vi "Module - Page Report.vi"(11 "Stop":bool) -> ()   [LabVIEW 2020]
uses:
  Control/State - eFGV.ctl
panel:
  in  "header name":T1={"Value 1"="", "Datetime"="Datetime", "Test Number"="Test Number", "Chart No"="Chart No", "Test Cycle"="Test Cycle", "Order Number"="Order Number", "Work Station"="Work Station", "Test Catergory"="Test Catergory", "Test Type"="Test Type", "Tested by"="Tested by", "Test Status"="Test Status", "Approved by TPI"="Approved by TPI"}
  in  "Table Report":T2(array[cluster])
  in  "Search 2":bool
  in  "Test Cycle":string(combo)
  in  "Test Type":string(combo)
  in  "Test Number":u16
  in  "Work Station":string(combo)
  in  "End Date":timestamp caption="To" format="%<%x %.3X>T"
  in  "Start Date":timestamp caption="Date" format="%<%x %.3X>T"
  in  "TPI Approval":bool
  in  "Overall Test Status":bool
  in  "Selection":string(combo)
  in  "Report Type":string(combo)
  # "REPORT"
  # "Approved Only"
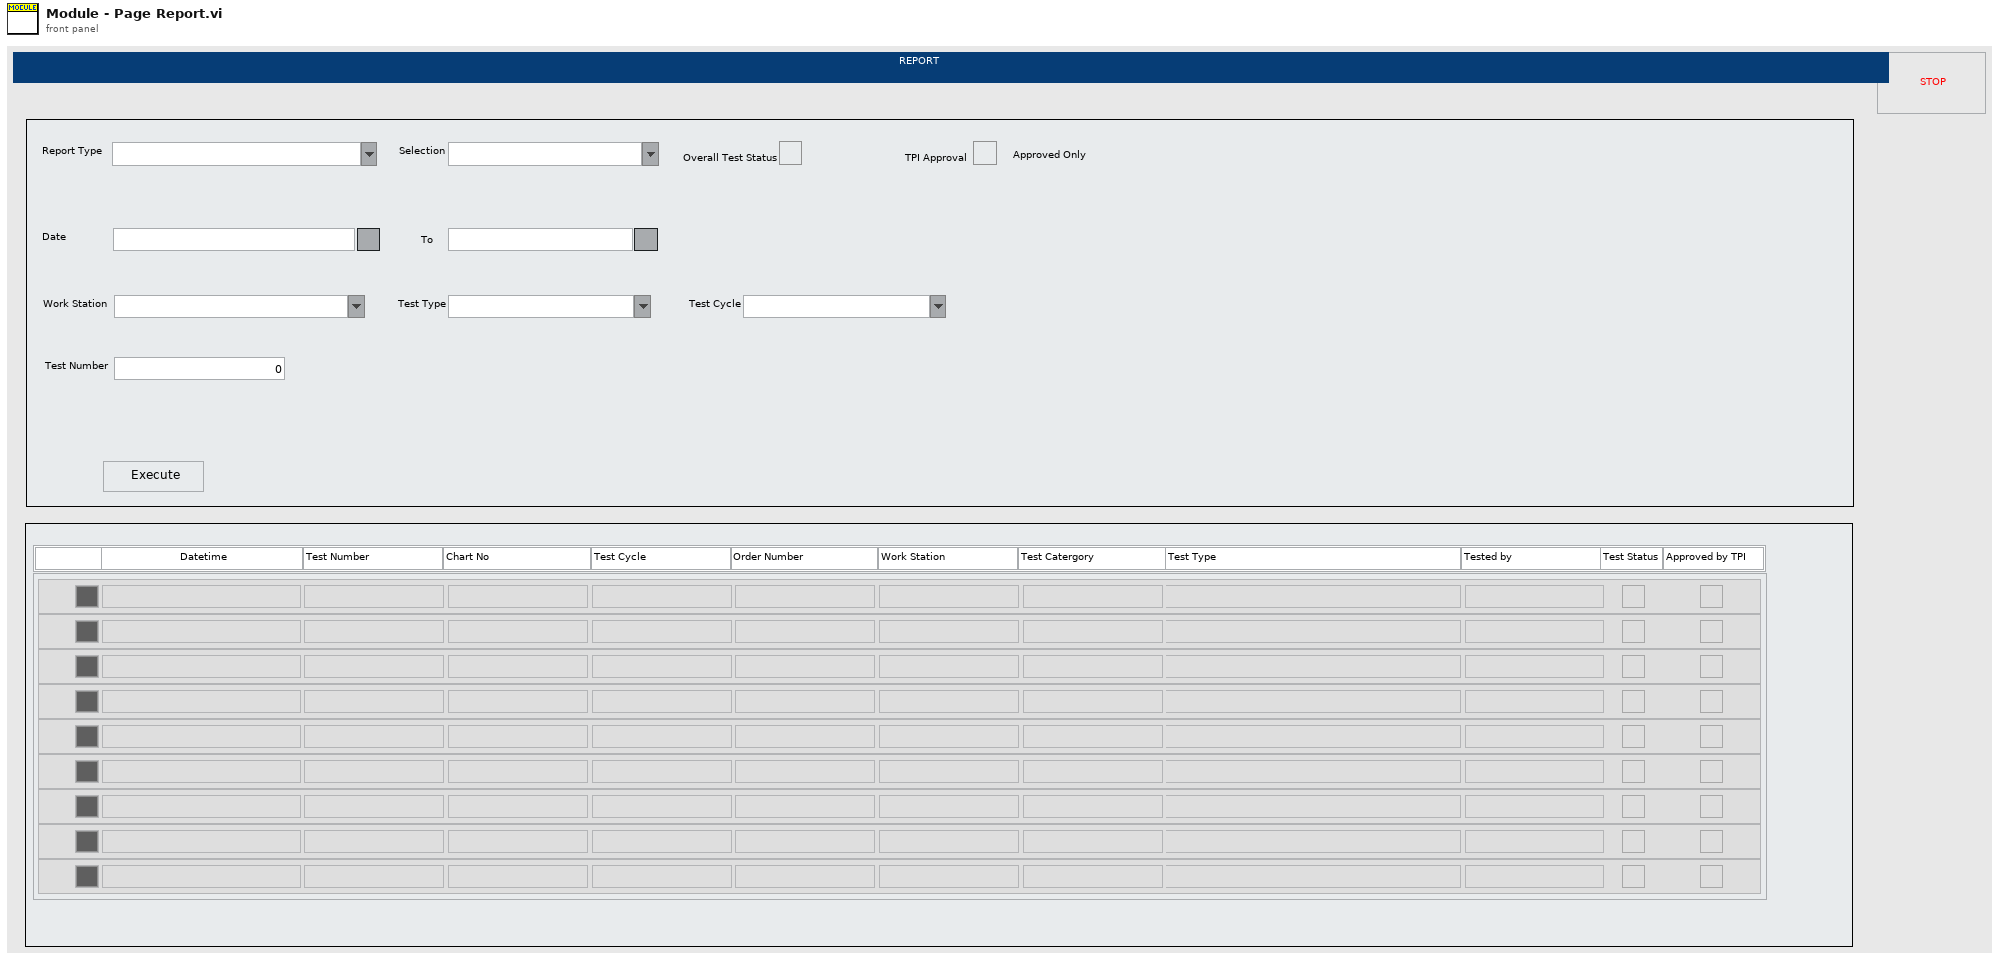
[diagram p1: front panel]
types:
  T1 = cluster{"Value 1":string, "Datetime":string, "Test Number":string, "Chart No":string, "Test Cycle":string, "Order Number":string, "Work Station":string, "Test Catergory":string, "Test Type":string, "Tested by":string, "Test Status":string, "Approved by TPI":string}
  T2 = cluster{"Datetime":string, "Test Number":string, "Test Cycle":string, "Chart No.":string, "Order Number":string, "Wortk Station ":string, "Test Category":string, "Test Type":string, "Test by":string, "Test Status":bool, "Approved by TPI":bool, "label":u32}[]
  T3 = cluster{"T_Out":i32, "Event Ref":refnum<event-registration>}
  T4 = enum16{"Init", "Register Event", "Idle", "Process", "Close"}
  T5 = typedef "State - eFGV.ctl" = enum16{"Init", "Read", "Write", "Exit"}
  T6 = enum32{"invalid app kind", "Development System", "Run Time System", "Student Edition", "Embedded LabVIEW", "Evaluation", "Custom"}
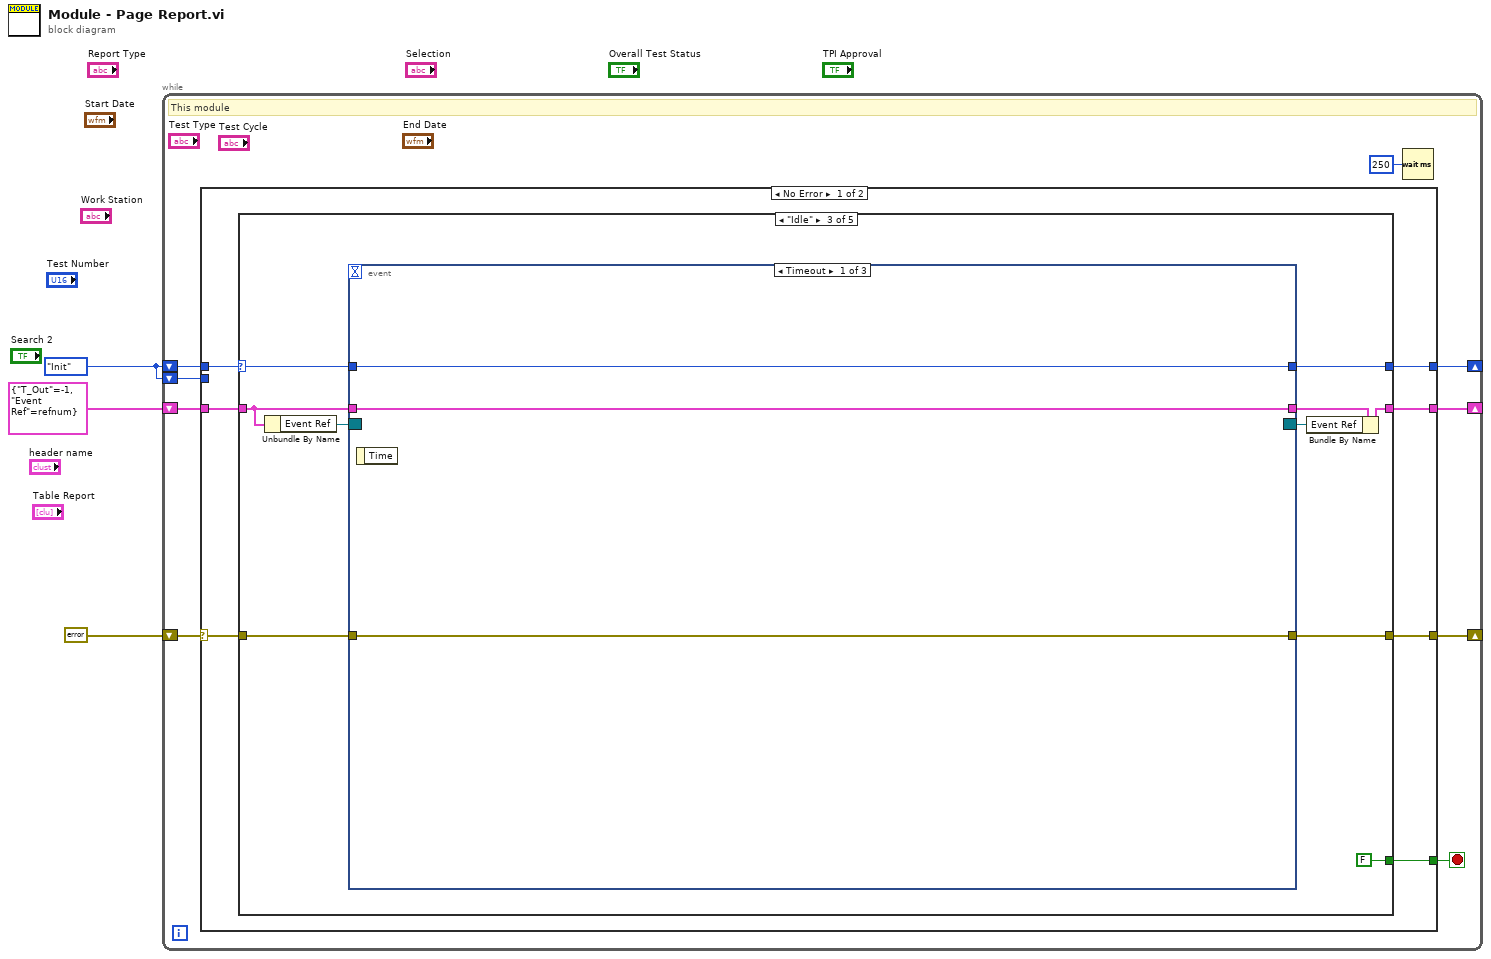
[diagram p0: block diagram]
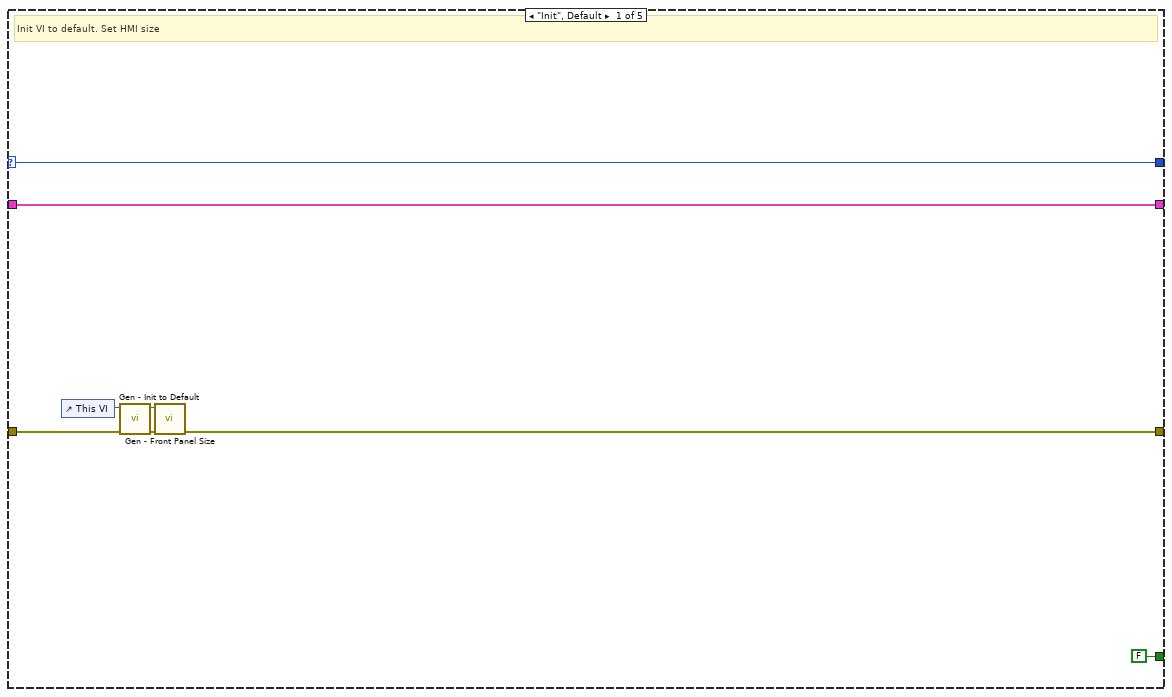
[diagram p2: hidden frame]
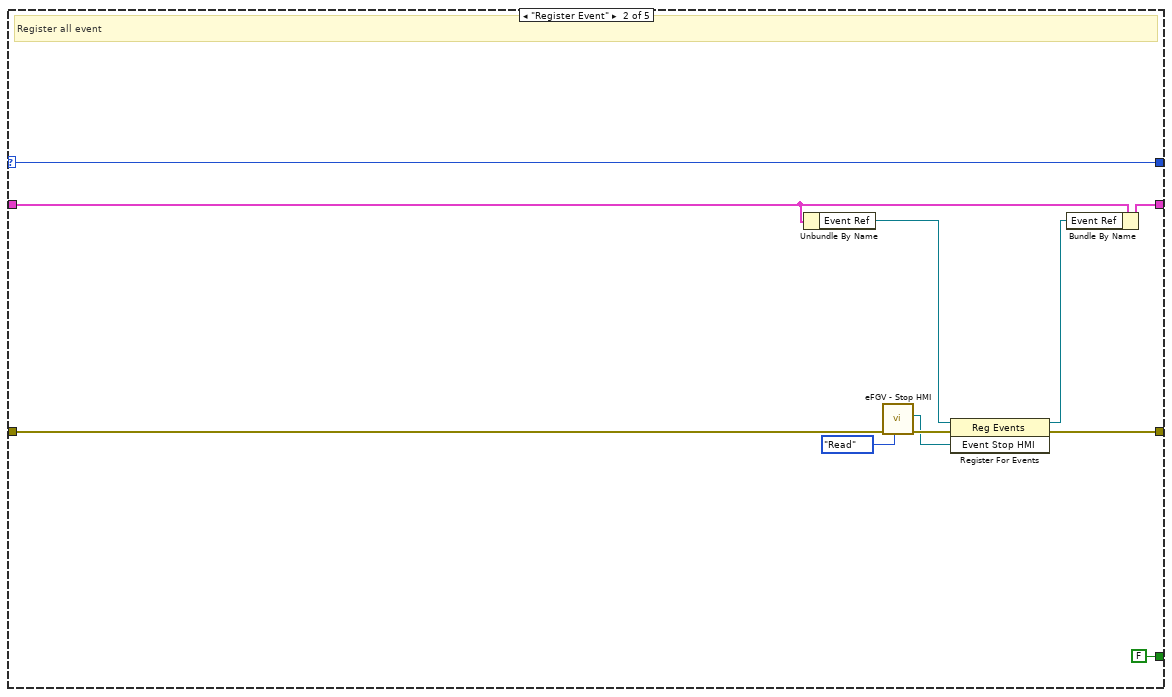
[diagram p3: hidden frame]
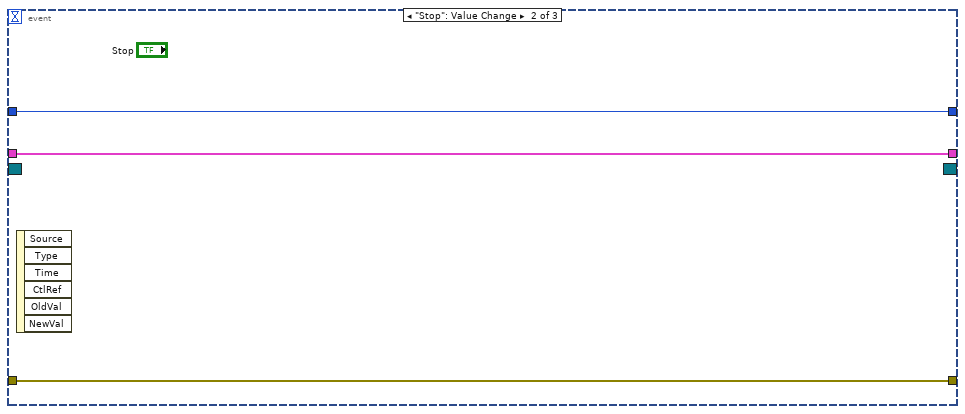
[diagram p4: hidden frame]
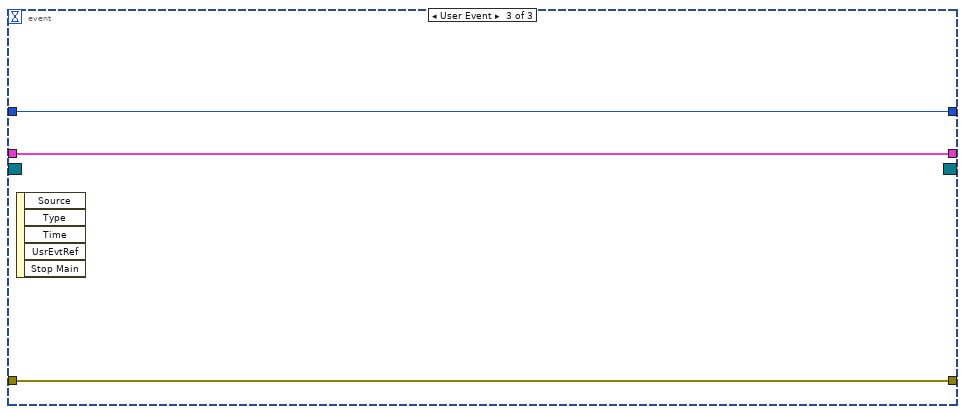
[diagram p5: hidden frame]
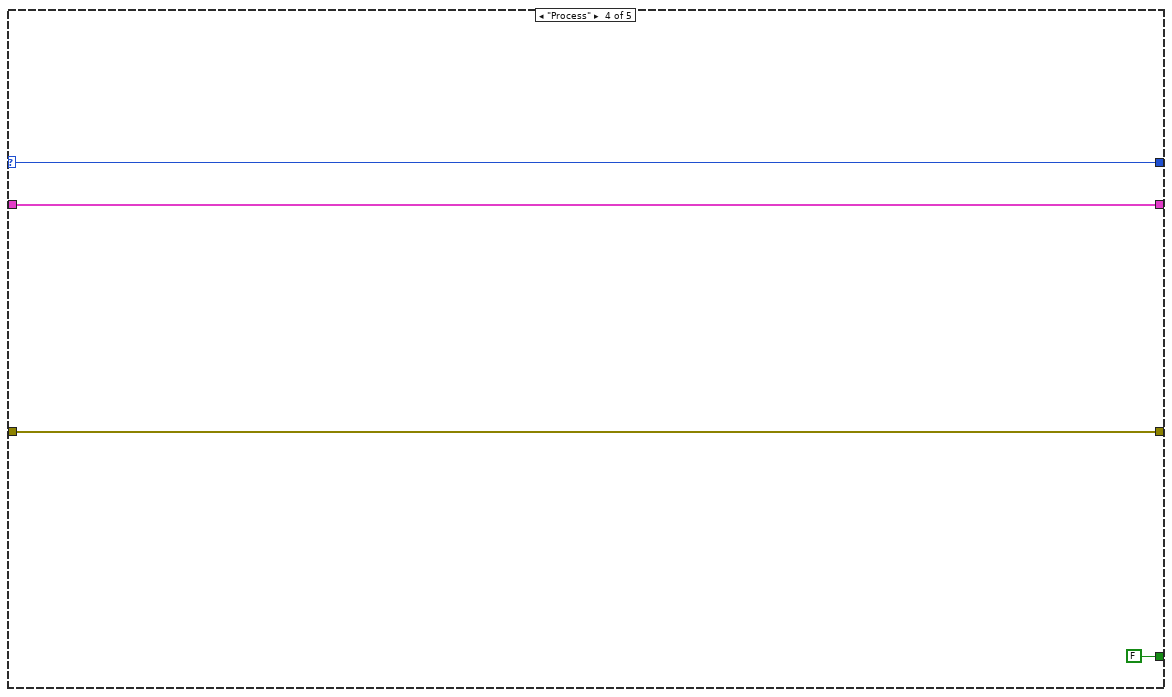
[diagram p6: hidden frame]
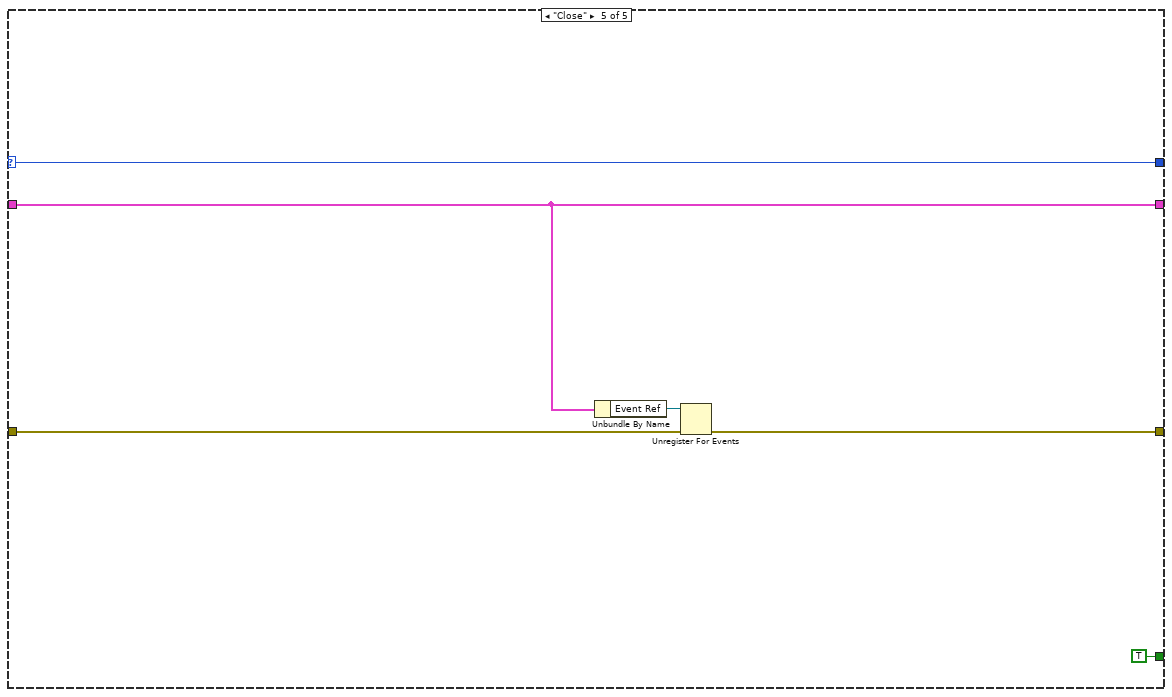
[diagram p7: hidden frame]
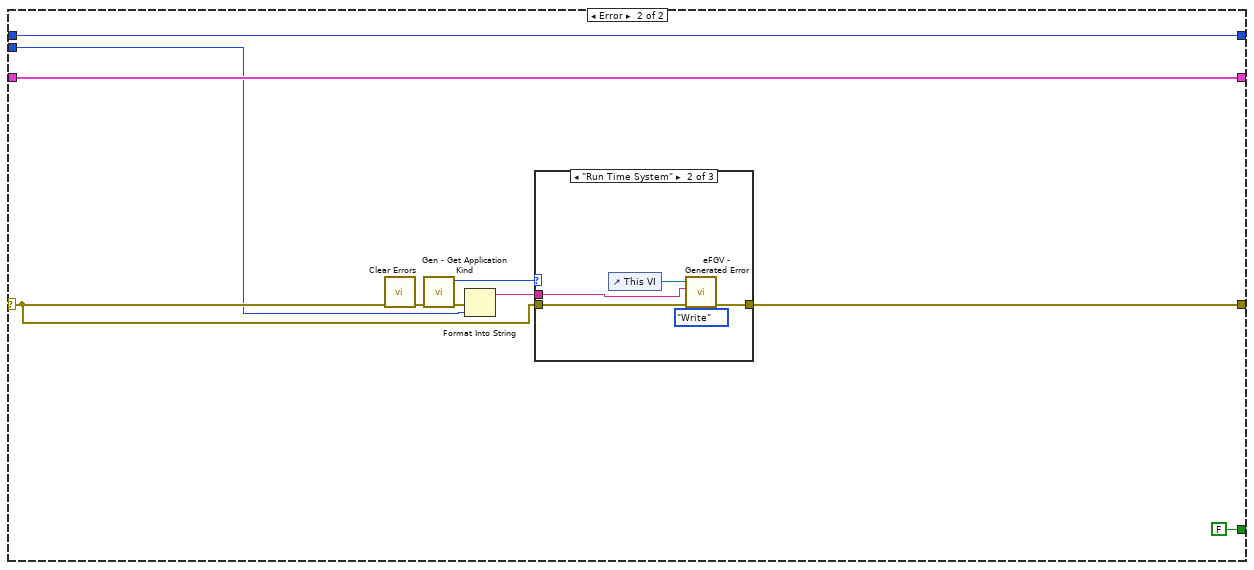
[diagram p8: hidden frame]
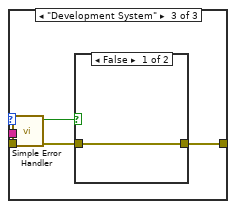
[diagram p10: hidden frame]
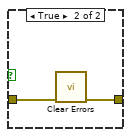
[diagram p11: hidden frame]
diagram:
  w1 = T4."Init"
  n1 = while {
    shift-right: [w8] -> _
    shift-left: w1 -> [w10]
    shift-right: [w11] -> _
    shift-left: errorcluster {"status"=FALSE, "code"=0, "source"=""} ("Error In") -> [w12]
    shift-right: [w6] -> _
    shift-left: T3 {"T_Out"=-1, "Event Ref"=refnum} -> [w7]
    shift-left: w1 -> [w4]
    stop <- w9 stop-if-true
    # "This module"
    n2 = case shown="No Error" w12 {
      selector: w12 -> [w18 w71]
      tunnel: w10 -> [w17 w76]
      tunnel: [w19 w72] -> w11
      tunnel: [w16 FALSE] -> w9
      tunnel: [w15 w76] -> w8
      tunnel: w7 -> [w14 w75]
      tunnel: [w13 w75] -> w6
      tunnel: w4 -> [_ w68]
      frame No Error {
        n3 = case shown="\"Idle\"" w17 {
          selector: w17 -> [w22 w34 w43 w58 w65]
          tunnel: [w25 w38 w48 w61 w66] -> w19
          tunnel: w18 -> [w27 w36 w47 w61 w67]
          tunnel: [FALSE FALSE FALSE FALSE TRUE] -> w16
          tunnel: [w22 w34 w45 w58 w65] -> w15
          tunnel: w14 -> [w24 w31 w42 w59 w63]
          tunnel: [w24 w29 w40 w59 w63] -> w13
          frame "Init", Default {
            # "Init VI to default. Set HMI size"
            n4 = control-ref of="This VI"() -> (w21:refnum<vi>)
            n5 = call "Gen - Init to Default.vi"("Error in"=w27, "This VI"=w21) -> ("Error out"=w26:errorcluster, "This VI Copy"=w20:refnum<vi>)  [unwired: 8 in]
            n6 = call "Gen - Front Panel Size.vi"("Error In"=w26, "This VI"=w20) -> ("Error Out"=w25:errorcluster)  [unwired: 9 in]
          }
          frame "Register Event" {
            # "Register all event"
            n7 = Unbundle By Name(w31) -> ("Event Ref"=w30:refnum<event-registration>)
            n8 = call "eFGV - Stop HMI.vi"("Action"=State_-_eFGV."Read", "Error In"=w36) -> ("Error Out"=w37:errorcluster, "Event Stop HMI"=w33:refnum<user-event>)  [unwired: 7 in, 1 out]
            n9 = register-events(reference=w30, error in=w37, w33) -> (reference out=w28:refnum<event-registration>, error out=w38:errorcluster)
            n10 = Bundle By Name(cluster=w31, "Event Ref"=w28) -> (w29:T3)
          }
          frame "Idle" {
            n11 = Unbundle By Name(w42) -> ("Event Ref"=w41:refnum<event-registration>)
            n12 = event shown="[0] Timeout" {
              selector: w41 -> [_ _ _]
              dyn-events: [_ _ _] -> w39
              timeout: _ -> [_ _ _]
              tunnel: [w49 w54 w57] -> w48
              tunnel: w47 -> [w49 w54 w57]
              tunnel: [w50 w52 w55] -> w45
              tunnel: [w51 w53 w56] -> w44
              tunnel: w42 -> [w51 w53 w56]
              tunnel: w43 -> [w50 w52 w55]
              event Timeout {
                n13 = event-data() -> ()  [unwired: 1 in, 1 out]
              }
              event "Stop": Value Change {
                n14 = event-data() -> ()  [unwired: 1 in, 6 out]
              }
              event User Event {
                n15 = event-data() -> ()  [unwired: 1 in, 5 out]
              }
            }
            n16 = Bundle By Name(cluster=w44, "Event Ref"=w39) -> (w40:T3)
          }
          frame "Process" {
          }
          frame "Close" {
            n17 = Unbundle By Name(w63) -> ("Event Ref"=w62:refnum<event-registration>)
            n18 = Unregister For Events(event registration refnum=w62, error in=w67) -> (error out=w66:errorcluster)
          }
        }
      }
      frame Error {
        n19 = call <vilib>:"Clear Errors.vi"("error in (no error)"=w71) -> ("error out"=w74:errorcluster)  [unwired: 5 in, 1 out]
        n20 = call "Gen - Get Application Kind.vi"("Error In"=w74) -> ("Error Out"=w70:errorcluster, "Application:Kind"=w73:T6)  [unwired: 9 in]
        n21 = Format Into String(error in=w70, w68) -> (resulting string=w69:string)  [unwired: 2 in, 1 out]
        n22 = case shown="\"Run Time System\"" w73 {
          tunnel: [w78 w83 w87] -> w72
          tunnel: w71 -> [w78 w80 w85]
          tunnel: w69 -> [_ w79 _]
          frame "invalid app kind", Default {
          }
          frame "Run Time System" {
            n23 = control-ref of="This VI"() -> (w81:refnum<vi>)
            n24 = call "eFGV - Generated Error.vi"("eFGV States"=State_-_eFGV."Write", "Error In"=w80, "State"=w79, "This VI"=w81) -> ("Error Out"=w83:errorcluster)  [unwired: 6 in, 1 out]
          }
          frame "Development System" {
            n25 = call <vilib>:"Simple Error Handler.vi"("error in (no error)"=w85) -> ("error?"=w84:bool, "error out"=w86:errorcluster)  [unwired: 4 in, 3 out]
            n26 = case shown="False" w84 {
              tunnel: [w88 w90] -> w87
              tunnel: w86 -> [w88 w89]
              frame False {
              }
              frame True {
                n27 = call <vilib>:"Clear Errors.vi"("error in (no error)"=w89) -> ("error out"=w90:errorcluster)  [unwired: 5 in, 1 out]
              }
            }
          }
        }
      }
    }
    n28 = Wait (ms)(milliseconds to wait=u32 250) -> ()  [unwired: 1 out]
  }
